vi "Extract Data1D.vi"(8 "error in (no error)":errorcluster, 10 "Data1D in":refnum<class "Data1D.lvclass">, 11 "MassSpectrumExtractor in":refnum<class "MassSpectrumExtractor.lvclass">) -> (0 "error out":errorcluster, 3 "MassSpectrumExtractor out":refnum<class "MassSpectrumExtractor.lvclass">)   [LabVIEW 2014, in "MassSpectrumExtractor.lvclass"]
uses:
  MassSpectrumExtractor.lvclass
  Framework/Model/Data/Data1D/Data1D.lvclass
  Framework/Model/Data/DataSingleElement/DataSingleElement.lvclass
  MassSpectrumExtractor.lvclass/MassSpectrumExtractor.ctl
  Graph with cursors/Graph with cursors XControl.xctl
  Framework/Interfaces/Observable Actor/Observable Actor.lvclass
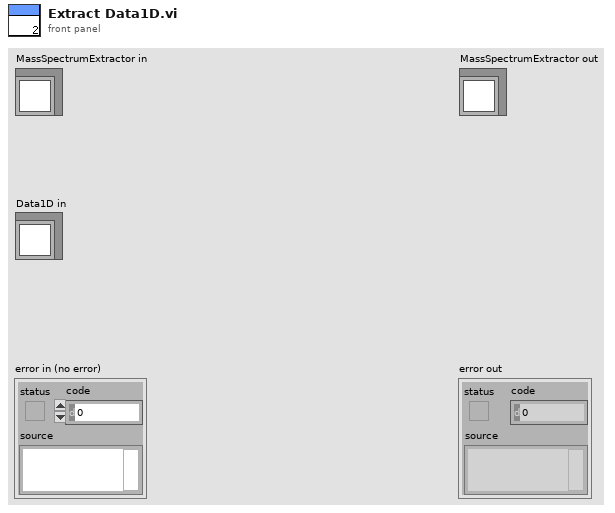
[diagram p1: front panel]
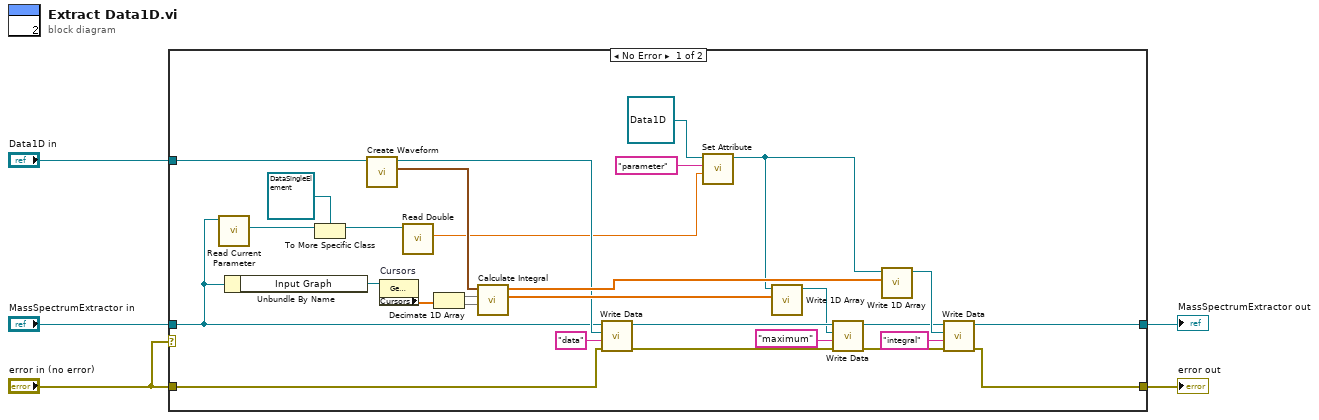
[diagram p0: block diagram]
diagram:
  n1 = case shown="No Error" "error in (no error)" {
    tunnel: "error in (no error)" -> [w22 w34]
    tunnel: [w24 w34] -> w5
    tunnel: "MassSpectrumExtractor in" -> [w10 w35]
    tunnel: [w15 w35] -> w3
    tunnel: "Data1D in" -> [w30 _]
    frame No Error {
      n2 = call-dynamic "Read Current Parameter.vi"("AbstractExtractor in"=w10) -> ("AbstractData.lvclass"=w9:refnum<class "AbstractData.lvclass">)  [unwired: 8 in, 2 out]
      n3 = Unbundle By Name(w10) -> ("Input Graph"=w28:refnum<vi>)
      n4 = To More Specific Class(target class=refnum<class "DataSingleElement.lvclass"> refnum ("DataSingleElement.lvclass"), reference=w9) -> (specific class reference=w7:refnum<class "DataSingleElement.lvclass">)  [unwired: 1 in, 1 out]
      n5 = call "Create Waveform.vi"("Data1D in"=w30) -> ("Waveform"=w31:waveform(dbl), "Data1D out"=w14:refnum<class "Data1D.lvclass">)  [unwired: 8 in, 1 out]
      n6 = property on="Cursors" class="Gen (strict)"(reference=w28) -> ("Cursors"=w27:dbl[])  [unwired: 1 in, 2 out]
      n7 = call "Read Double.vi"("DataSingleElement in"=w7) -> ("value"=w6:dbl)  [unwired: 8 in, 2 out]
      n8 = Decimate 1D Array(w27) -> (w32:dbl[], w33:dbl[])
      n9 = call "Calculate Integral.vi"("Right Boundary Array"=w33, "Left Boundary Array"=w32, "Waveform"=w31) -> ("Maximums"=w20:dbl[], "Integrals"=w29:dbl[])  [unwired: 7 in]
      n10 = call "Write Data.vi"("error in (no error)"=w22, "Name"="data", "Data"=w14, "Observable Actor in"=w10) -> ("error out"=w21:errorcluster, "Observable Actor out"=w18:refnum<class "MassSpectrumExtractor.lvclass">)  [unwired: 6 in]
      n11 = call-dynamic "Set Attribute.vi"("Value"=w6, "Name"="parameter", "AbstractData in"=refnum<class "Data1D.lvclass"> refnum ("Data1D.lvclass")) -> ("AbstractData out"=w13:refnum<class "Data1D.lvclass">)  [unwired: 6 in, 2 out]
      n12 = call "Write 1D Array.vi"("1D Array"=w20, "Data1D in"=w13) -> ("Data1D out"=w16:refnum<class "Data1D.lvclass">)  [unwired: 8 in, 1 out]
      n13 = call "Write Data.vi"("Name"="maximum", "Data"=w16, "Observable Actor in"=w18) -> ("Observable Actor out"=w17:refnum<class "MassSpectrumExtractor.lvclass">)  [unwired: 7 in, 1 out]
      n14 = call "Write 1D Array.vi"("1D Array"=w29, "Data1D in"=w13) -> ("Data1D out"=w26:refnum<class "Data1D.lvclass">)  [unwired: 8 in, 1 out]
      n15 = call "Write Data.vi"("error in (no error)"=w21, "Name"="integral", "Data"=w26, "Observable Actor in"=w17) -> ("error out"=w24:errorcluster, "Observable Actor out"=w15:refnum<class "MassSpectrumExtractor.lvclass">)  [unwired: 6 in]
    }
    frame Error {
    }
  }
  "error out" <- w5
  "MassSpectrumExtractor out" <- w3
